vi "Test_Spectrum_With_Accums.vi"(8 "error in (no error)":errorcluster) -> (0 "error out":errorcluster)   [LabVIEW 2015]
doc: "This VI inits a waveform generation session for AWG-5421. This is a basic example that shows how to setup the board in order to generate waveforms according to a script. \nBy default this configuration uses one channel CH0, and one script trigger ScriptTrigger0. The ScriptTrigger0 is waiting for an external trigger : i.e. a digital Edge on pin PFI 0 by default.\n\nThere are various options for the script to be used. Consult the Script control help for more information on configuring the example for specific scripts."
uses:
  controls/SOFTWARE_Inputs.ctl
panel:
  in  "Accumulations":i32=1
  out "Current Spectrum":path
  in  "SOFTWARE Inputs":T1={"Application Directory"=path "D:/S.O.F.T.S/LABVIEW/PIL", "Resources Path"=path "D:/S.O.F.T.S/LABVIEW/PIL/resources", "Data Path"=path "D:/PIRENEA/DATA", "XML Path"=path "D:/PIRENEA/DATA", "XML File Filter"="*.xml", "Excit Scripts Path"=path "D:/PIRENEA/EXCIT_SCRIPTS", "Excit Scripts File Filter"="*.txt", "Excit Waveforms Path"=path "D:/PIRENEA/EXCIT_WFMS", "Excit Waveforms File Filter"="*.bin", "Timing Scripts Path"=path "D:/PIRENEA/TIMING_SCRIPTS", "Timing Scripts File Filter"="*.txt", "Timing Waveforms Path"=path "D:/PIRENEA/TIMING_WFMS", "Timing Waveforms File Filter"="*.bin", "Trapping Waveforms Path"=path "D:/PIRENEA/TRAPPING_WFMS", "Trapping Waveforms File Filter"="*.bin"}
  in  "chemin du fichier (utiliser une boîte de dialogue)":path=path "D:/PIRENEA/DATA/2016/data_2016_11_22/2016_11_22_016.A00"
  out "Data Size (samples)":i32
  out "Total Size (bytes)":i64
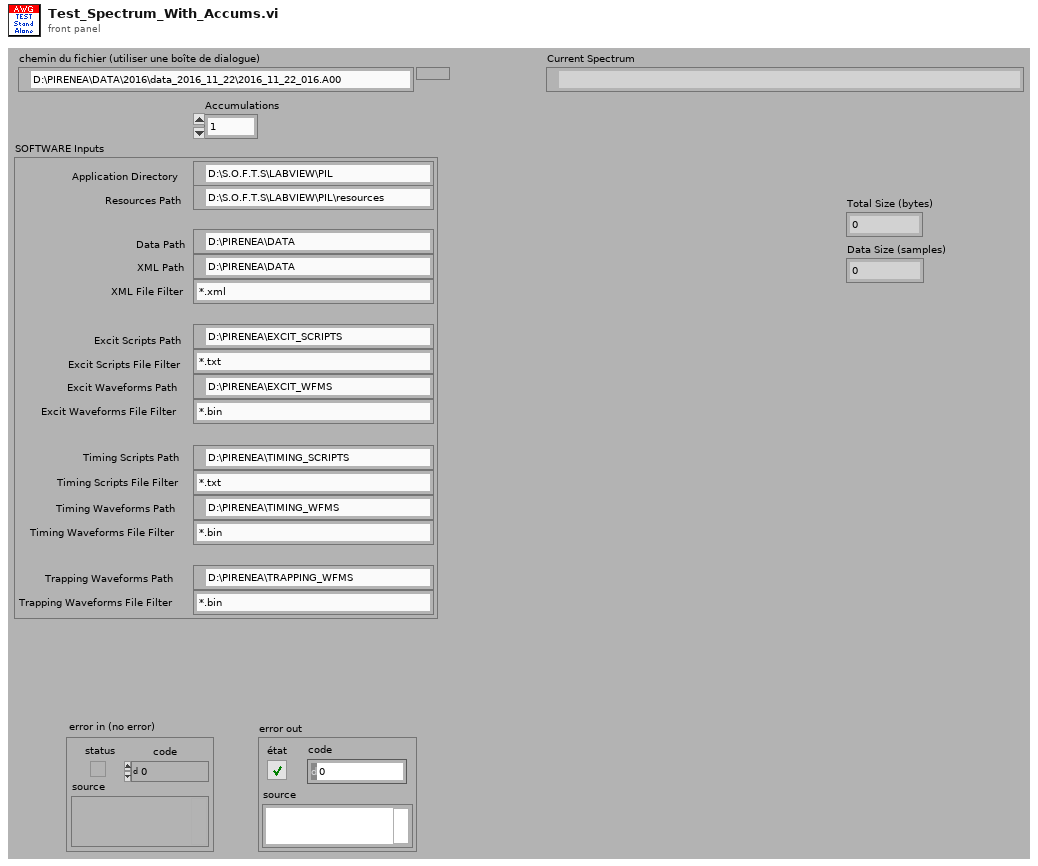
[diagram p1: front panel]
types:
  T1 = typedef "SOFTWARE_Inputs.ctl" = cluster{"Application Directory":path, "Resources Path":path, "Data Path":path, "XML Path":path, "XML File Filter":string, "Excit Scripts Path":path, "Excit Scripts File Filter":string, "Excit Waveforms Path":path, "Excit Waveforms File Filter":string, "Timing Scripts Path":path, "Timing Scripts File Filter":string, "Timing Waveforms Path":path, "Timing Waveforms File Filter":string, "Trapping Waveforms Path":path, "Trapping Waveforms File Filter":string}
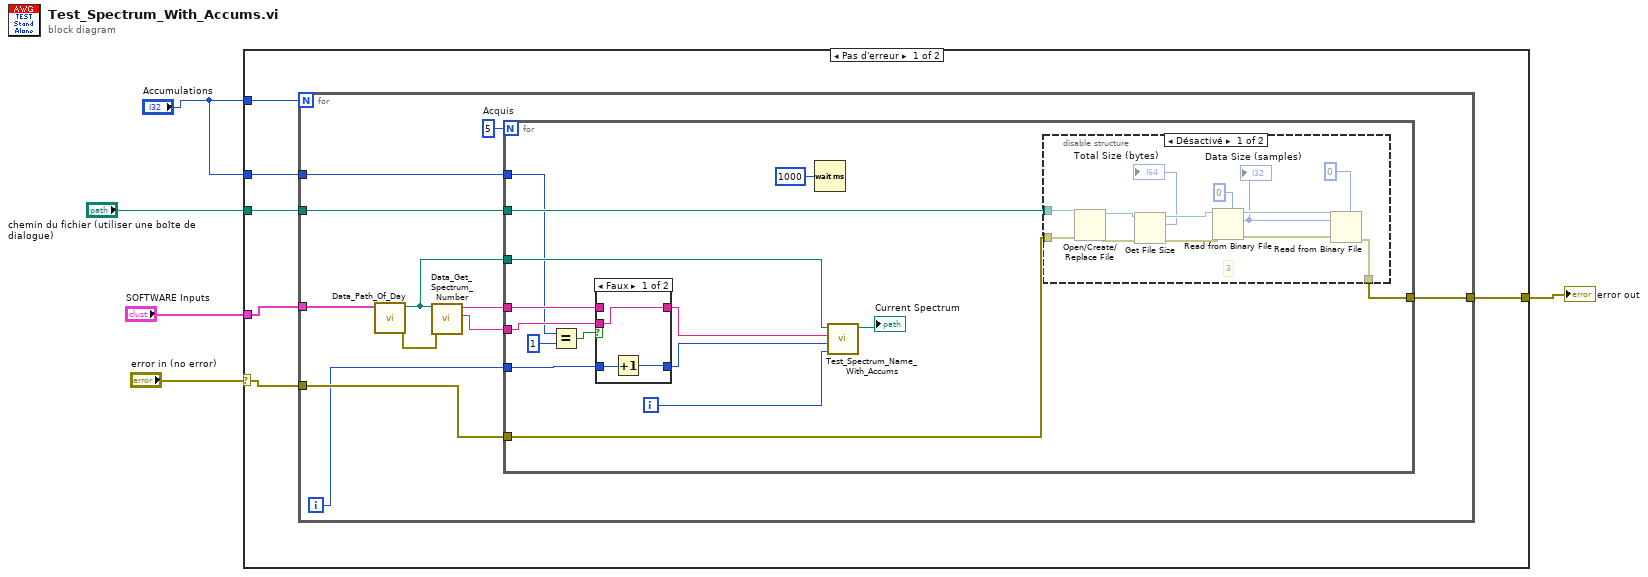
[diagram p0: block diagram]
diagram:
  n1 = case shown="Pas d'erreur" "error in (no error)" {
    selector: "error in (no error)" -> [w11 w56]
    tunnel: "chemin du fichier (utiliser une boîte de dialogue)" -> [w10 _]
    tunnel: "SOFTWARE Inputs" -> [w9 _]
    tunnel: [w8 w56] -> w2
    tunnel: "Accumulations" -> [w7 _]
    tunnel: "Accumulations" -> [w6 _]
    frame No Error {
      n2 = for {
        N: w7 -> [_]
        tunnel: w11 -> [w22]
        tunnel: w10 -> [w21]
        tunnel: w9 -> [w18]
        tunnel: [w14] -> w8
        tunnel: w6 -> [w12]
        i -> [w15]
        w20 = 5  # Acquis
        n3 = call "Data_Path_Of_Day.vi"("SOFTWARE Inputs"=w18) -> ("error out"=w19:errorcluster, "Path of the Day"=w16:path)  [unwired: 9 in]
        n4 = call "Data_Get_Spectrum_Number.vi"("error in (no error)"=w19, "Path of the Day"=w16) -> ("Last Spectrum Number"=w13:string, "Next Spectrum Number"=w17:string)  [unwired: 7 in, 1 out]
        n5 = for {
          N: w20 -> [_]
          tunnel: w22 -> [w37]
          tunnel: w21 -> [w36]
          tunnel: w17 -> [w31]
          tunnel: w16 -> [w35]
          tunnel: w15 -> [w29]
          tunnel: [w33] -> w14
          tunnel: w13 -> [w32]
          tunnel: w12 -> [w25]
          i -> [w23]
          n6 = Equal?(x=w25, y=1) -> (x = y?=w27:bool)
          n7 = case shown="Faux" w27 {
            tunnel: w32 -> [w53 _]
            tunnel: w31 -> [_ w55]
            tunnel: [w53 w55] -> w30
            tunnel: w29 -> [w52 w54]
            tunnel: [w51 w54] -> w28
            frame False {
              n8 = Increment(x=w52) -> (x+1=w51:i32)
            }
            frame True {
            }
          }
          n9 = Wait (ms)(milliseconds to wait=u32 1000 ("attente (ms)")) -> ()  [unwired: 1 out]
          n10 = call "Test_Spectrum_Name_With_Accums.vi"("Acquis Number"=w23, "Accum Number"=w28, "Next Spectrum Number"=w30, "Path of the Day"=w35) -> ("chemin complet"=→"Current Spectrum":path)  [unwired: 7 in]
          n11 = disable-structure shown="Désactivé" {
            disable-tunnel: w37 -> [w41 _]
            disable-tunnel: w36 -> [w40 _]
            disable-tunnel: [w38 _] -> w33
            frame Disabled {
              # "3"
              n12 = Open/Create/Replace File(file path (use dialog)=w40, error in=w41) -> (refnum out=w49:refnum<file>, error out=w48:errorcluster)  [unwired: 4 in, 1 out]
              n13 = Get File Size(file=w49, error in=w48) -> (refnum out=w47:refnum<file>, size (in bytes)=→"Total Size (bytes)":i64, 0:w46:errorcluster)
              n14 = Read from Binary File(5:0, 8:w46, 11:w47) -> (0:w43:errorcluster, 2:w39:i32, 3:w44:refnum<file>)  [unwired: 3 in, 1 out]
              "Data Size (samples)" <- w39
              n15 = Read from Binary File(5:i16 0, 8:w43, 10:w39, 11:w44) -> (0:w38:errorcluster)  [unwired: 2 in, 3 out]
            }
            frame Enabled {
            }
          }
        }
      }
    }
    frame Error {
    }
  }
  "error out" <- w2
